vi "CFN61G_B89-90-to-Cluster_v1.vi"(11 "Align_Word":u16) -> (3 "Cluster":T1)   [LabVIEW 2017]
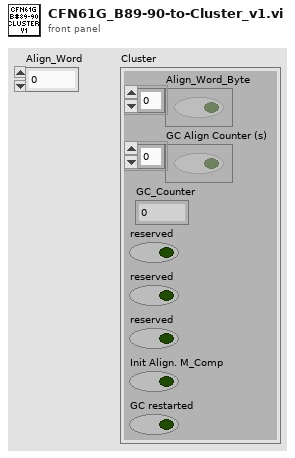
[diagram p1: front panel]
types:
  T1 = cluster{"Align_Word_Byte":bool[], "GC Align Counter (s)":bool[], "GC_Counter":u32, "reserved":bool, "reserved":bool, "reserved":bool, "Init Align. M_Comp":bool, "GC restarted ":bool}
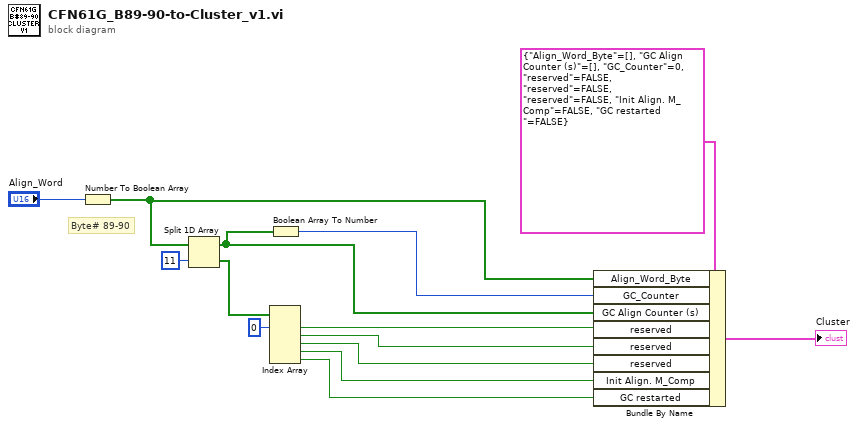
[diagram p0: block diagram]
diagram:
  # "Byte# 89-90"
  n1 = Number To Boolean Array(number="Align_Word") -> (Boolean array=w7:bool[])
  n2 = Split 1D Array(array=w7, index=11) -> (first subarray=w9:bool[], second subarray=w3:bool[])
  n3 = Index Array(array=w3, index #1=0 ("index")) -> (element #1=w10:bool, element #2=w11:bool, element #3=w12:bool, element #4=w13:bool, element #5=w14:bool)  [unwired: 4 in]
  n4 = Boolean Array To Number(Boolean array=w9) -> (number=w8:u32)
  n5 = Bundle By Name(cluster=T1 {"Align_Word_Byte"=[], "GC Align Counter (s)"=[], "GC_Counter"=0, "reserved"=FALSE, "reserved"=FALSE, "reserved"=FALSE, "Init Align. M_Comp"=FALSE, "GC restarted "=FALSE}, "Align_Word_Byte"=w7, "GC_Counter"=w8, "GC Align Counter (s)"=w9, "reserved"=w10, "reserved"=w11, "reserved"=w12, "Init Align. M_Comp"=w13, "GC restarted"=w14) -> (→"Cluster":T1)
